vi "Indices of Negative Array Elements.vi"(1 "Array In":dbl[](array[numeric])) -> (0 "Indices":i32[](array[numeric]))   [LabVIEW 2020]
doc: "Indices of Negative Array Elements.vi outputs an integer array containing the indices of any negative elements of the inputted double numeric array."
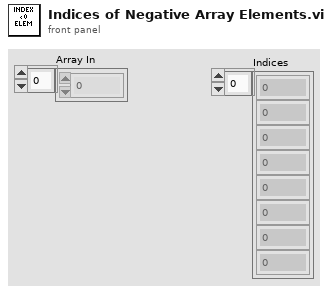
[diagram p1: front panel]
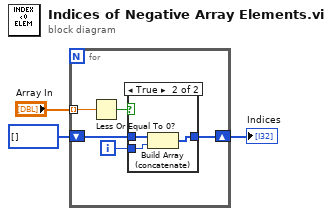
[diagram p0: block diagram]
diagram:
  n1 = for {
    tunnel: "Array In" -> [w8] mode=indexing
    shift-right: [w5] -> w1
    shift-left: i32[] [] -> [w4]
    i -> [w6]
    n2 = Less Or Equal To 0?(x=w8) -> (x <= 0?=w7:bool)
    n3 = case shown="True" w7 {
      tunnel: w6 -> [_ w10]
      tunnel: [w9 w12] -> w5
      tunnel: w4 -> [w9 w11]
      frame False {
      }
      frame True {
        n4 = Build Array (concatenate)(w11, w10) -> (w12:i32[])
      }
    }
  }
  "Indices" <- w1
